vi "Example.vi"() -> ()   [LabVIEW 2023]
uses:
  BS6006PRPLUS.lvlib
panel:
  out "Serial Number":string
  in  "Pulse":u16(ring)=2 items=["-25 V  0.1 uJ DC-20 MHz", "-45 V  0.4 uJ  DC - 30 MHz", "-75 V  1.0 uJ  DC - 35 MHz", "-120 V  2.4 uJ  DC - 45 MHz", "-190 V  5.0 uJ  DC - 50 MHz", "-190 V  11 uJ  DC - 25 MHz", "-190 V  15 uJ  DC - 20 MHz", "-190 V  20 uJ  DC - 15 MHz", "-190 V  25 uJ  DC - 12 MHz", "-190 V  30 uJ  DC - 10 MHz", "-190 V  35 uJ  DC - 9 MHz", "-190 V  40 uJ  DC - 8 MHz", "-190 V  45 uJ  DC - 7 MHz", "-190 V  50 uJ  DC - 6 MHz"]
  in  "PRF (Hz)":u16(ring)=200 items=["100"=100, "200"=200, "500"=500, "1000"=1000, "2000"=2000, "5000"=5000, "10000"=10000]
  in  "End":bool
  out "Waveform Graph":dbl[][](graph)
  in  "Number of Signals to be Acquired":i32
  in  "Length of Signal":i32
  in  "Enable Waveform Acquisition":bool
  in  "Stop":bool
  in  "Run":bool
  in  "Trigger Source":u16(ring) items=["Internal", "External"]
  in  "Mode":u16(ring) items=["ECHO", "THRU"]
  in  "Gain":i32
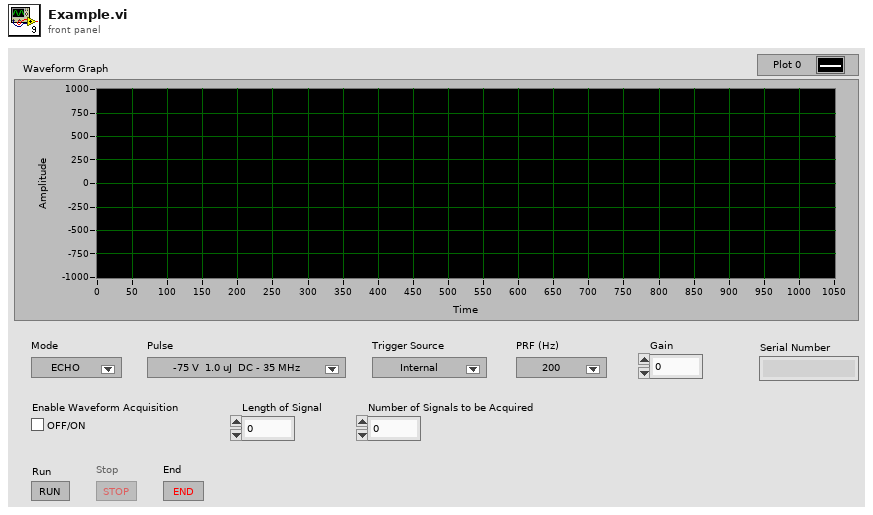
[diagram p1: front panel]
types:
  T1 = enum8{"Enabled", "Disabled", "Disabled and Grayed Out"}
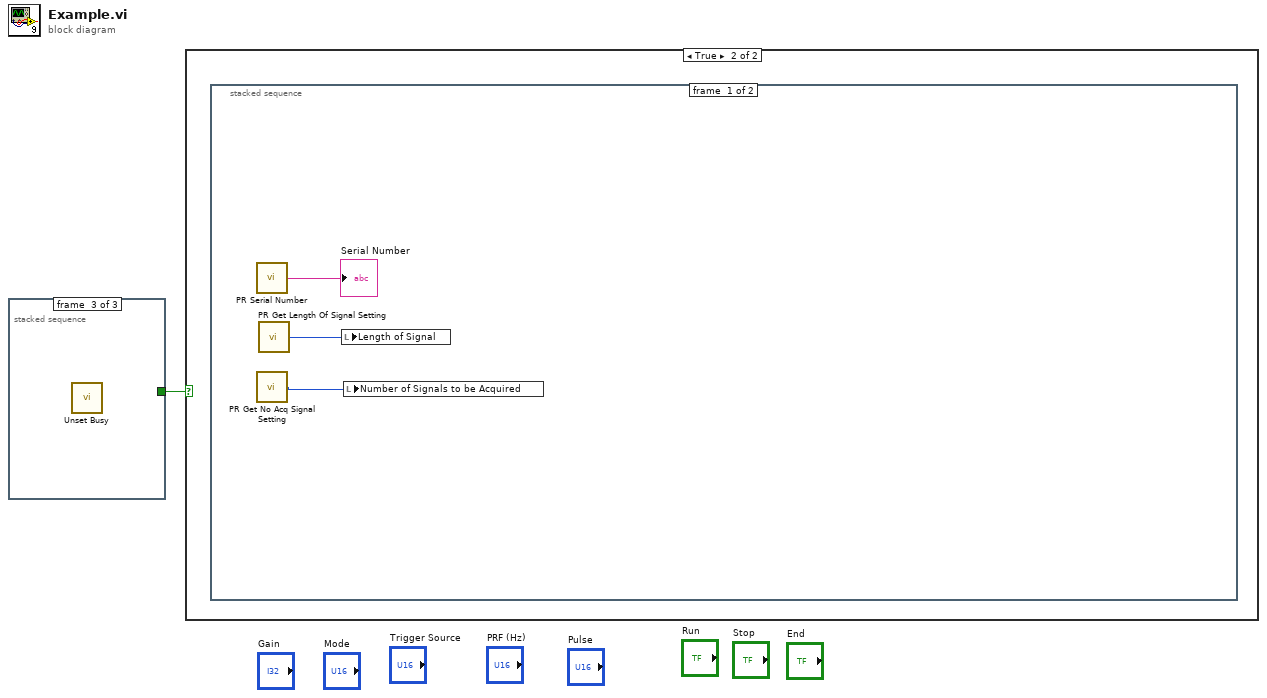
[diagram p0: block diagram]
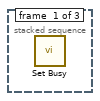
[diagram p2: hidden frame]
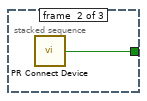
[diagram p3: hidden frame]
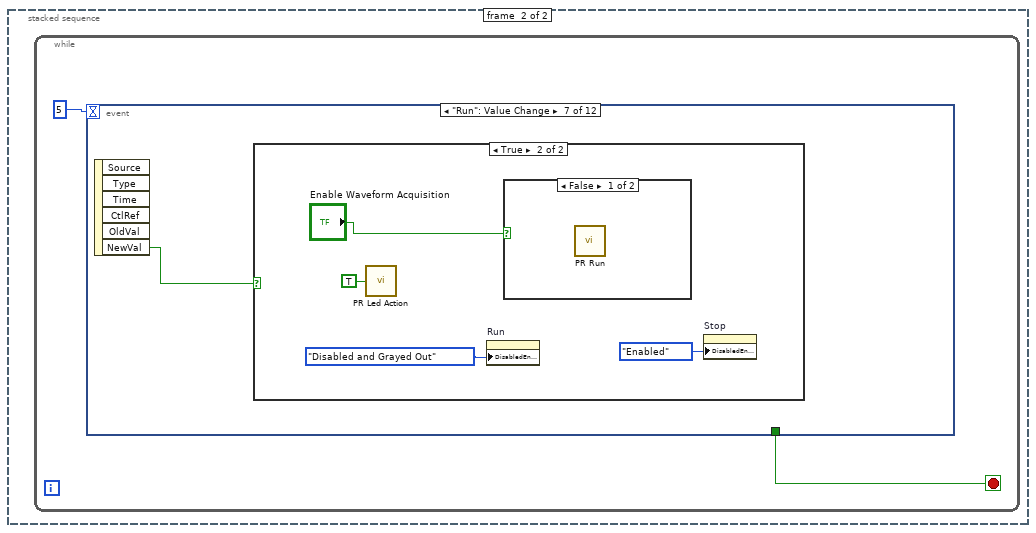
[diagram p5: hidden frame]
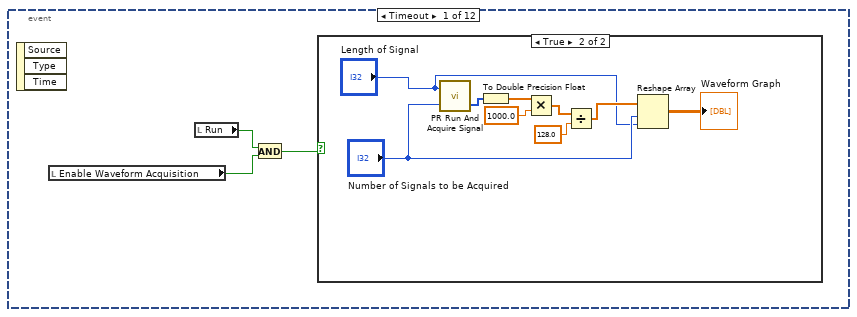
[diagram p6: hidden frame]
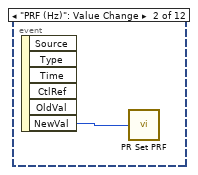
[diagram p8: hidden frame]
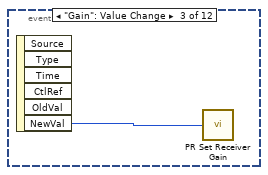
[diagram p9: hidden frame]
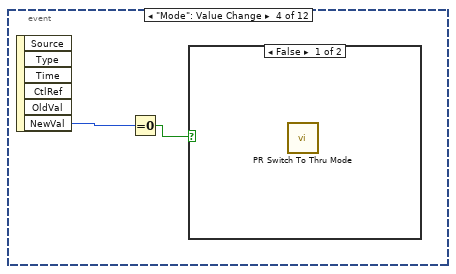
[diagram p10: hidden frame]
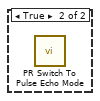
[diagram p11: hidden frame]
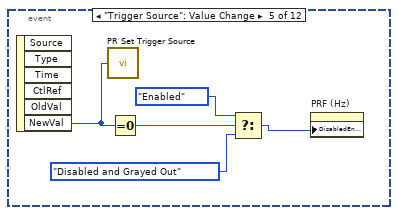
[diagram p12: hidden frame]
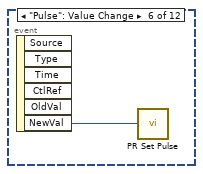
[diagram p13: hidden frame]
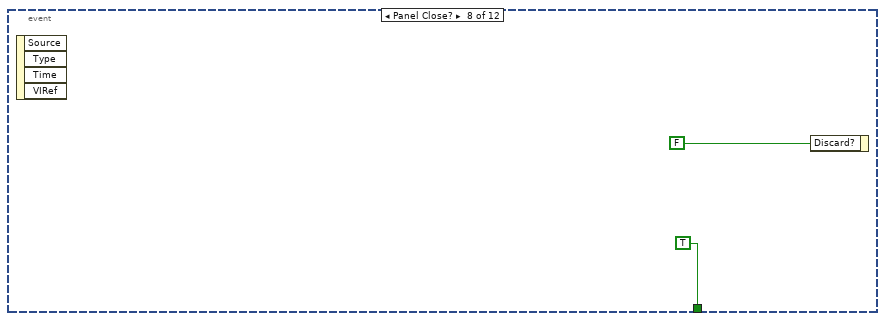
[diagram p16: hidden frame]
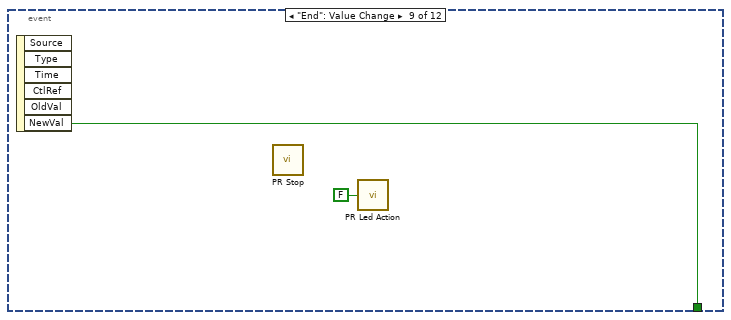
[diagram p17: hidden frame]
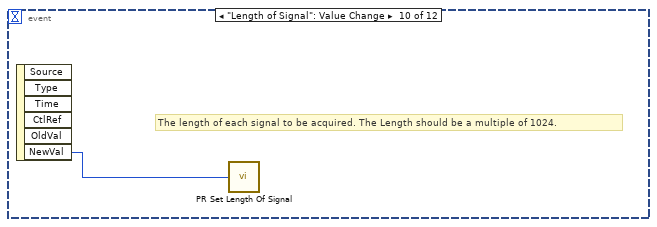
[diagram p18: hidden frame]
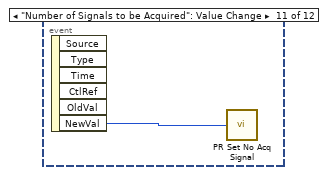
[diagram p19: hidden frame]
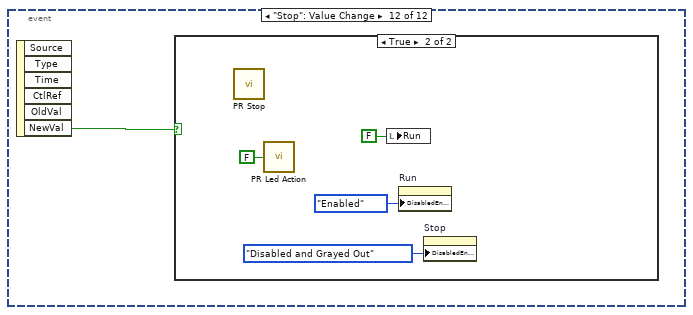
[diagram p20: hidden frame]
diagram:
  n1 = stacked-sequence {
    tunnel: [_ w2 _] -> w1
    frame #0 {
      n2 = call <vilib>:"Set Busy.vi"() -> ()  [unwired: 10 in, 2 out]
    }
    frame #1 {
      n3 = call "PR Connect Device.vi"() -> ("Connected"=w2:bool)
    }
    frame #2 {
      n4 = call <vilib>:"Unset Busy.vi"() -> ()  [unwired: 11 in, 1 out]
    }
  }
  n5 = case shown="True" w1 {
    frame False {
    }
    frame True {
      n6 = stacked-sequence {
        frame #0 {
          n7 = call "PR Serial Number.vi"() -> ("Serial Number"=→"Serial Number":string)
          n8 = call "PR Get No Acq Signal Setting.vi"() -> ("NoAcqSianglSetting"=w4:i32)
          n9 = call "PR Get Length Of Signal Setting.vi"() -> ("CurrentLength"=w5:i32)
          n10 = local write "Length of Signal"(w5) -> ()
          n11 = local write "Number of Signals to be Acquired"(w4) -> ()
        }
        frame #1 {
          n12 = while {
            stop <- w7 stop-if-true
            n13 = event shown="[6] \"Run\": Value Change" {
              selector: _ -> [_ _ _ _ _ _ _ _ _ _ _ _]
              dyn-events: _ -> [_ _ _ _ _ _ _ _ _ _ _ _]
              timeout: 5 -> [_ _ _ _ _ _ _ _ _ _ _ _]
              tunnel: [_ _ _ _ _ _ _ TRUE w38 _ _ _] -> w7
              event Timeout {
                n14 = event-data() -> ()  [unwired: 1 in, 3 out]
                n15 = local read "Enable Waveform Acquisition"() -> (w9:bool)
                n16 = local read "Run"() -> (w10:bool)
                n17 = And(x=w10, y=w9) -> (x .and. y?=w8:bool)
                n18 = case shown="True" w8 {
                  frame False {
                  }
                  frame True {
                    n19 = call "PR Run And Acquire Signal.vi"("Number of Signals to be Acquired"="Number of Signals to be Acquired", "Length of Signal"="Length of Signal") -> ("DataArray Out"=w19:i8[])  [unwired: 1 out]
                    n20 = To Double Precision Float(number=w19) -> (double precision float=w18:dbl[])
                    n21 = Multiply(x=w18, y=1000.0) -> (x*y=w16:dbl[])
                    n22 = Divide(x=w16, y=128.0) -> (x/y=w14:dbl[])
                    n23 = Reshape Array(w14, "Number of Signals to be Acquired", "Length of Signal") -> (→"Waveform Graph":dbl[][])
                  }
                }
              }
              event "PRF (Hz)": Value Change {
                n24 = event-data() -> ("NewVal"=w20:u16)  [unwired: 1 in, 5 out]
                n25 = call "PR Set PRF.vi"("PRF"=w20) -> ()  [unwired: 1 out]
              }
              event "Gain": Value Change {
                n26 = event-data() -> ("NewVal"=w21:i32)  [unwired: 1 in, 5 out]
                n27 = call "PR Set Receiver Gain.vi"("Gain"=w21) -> ()
              }
              event "Mode": Value Change {
                n28 = event-data() -> ("NewVal"=w23:u16)  [unwired: 1 in, 5 out]
                n29 = Equal To 0?(x=w23) -> (x = 0?=w22:bool)
                n30 = case shown="False" w22 {
                  frame False {
                    n31 = call "PR Switch To Thru Mode.vi"() -> ()  [unwired: 1 in]
                  }
                  frame True {
                    n32 = call "PR Switch To Pulse Echo Mode.vi"() -> ()  [unwired: 12 in]
                  }
                }
              }
              event "Trigger Source": Value Change {
                n33 = event-data() -> ("NewVal"=w28:u16)  [unwired: 1 in, 5 out]
                n34 = call "PR Set Trigger Source.vi"("TriggerSource"=w28) -> ()
                n35 = Equal To 0?(x=w28) -> (x = 0?=w27:bool)
                n36 = Select(t=T1."Enabled" ("Disabled"), s=w27, f=T1."Disabled and Grayed Out" ("Disabled")) -> (s? t:f=w24:T1)
                n37 = property on="PRF (Hz)" class="Ring (strict)"("DisabledEnum"=w24) -> ()  [unwired: 2 in, 2 out]
              }
              event "Pulse": Value Change {
                n38 = event-data() -> ("NewVal"=w29:u16)  [unwired: 1 in, 5 out]
                n39 = call "PR Set Pulse.vi"("PulseIndex"=w29) -> ()  [unwired: 1 out]
              }
              event "Run": Value Change {
                n40 = event-data() -> ("NewVal"=w30:bool)  [unwired: 1 in, 5 out]
                n41 = case shown="True" w30 {
                  frame False {
                  }
                  frame True {
                    n42 = call "PR Led Action.vi"("Enable"=TRUE) -> ()
                    n43 = property on="Run" class="Bool (strict)"("DisabledEnum"=T1."Disabled and Grayed Out" ("Disabled")) -> ()  [unwired: 2 in, 2 out]
                    n44 = case shown="False" "Enable Waveform Acquisition" {
                      frame False {
                        n45 = call "PR Run.vi"() -> ()  [unwired: 12 in]
                      }
                      frame True {
                      }
                    }
                    n46 = property on="Stop" class="Bool (strict)"("DisabledEnum"=T1."Enabled" ("Disabled")) -> ()  [unwired: 2 in, 2 out]
                  }
                }
              }
              event Panel Close? {
                n47 = event-data() -> ()  [unwired: 1 in, 4 out]
                n48 = event-data("Discard?"=FALSE) -> ()  [unwired: 1 in, 1 out]
              }
              event "End": Value Change {
                n49 = event-data() -> ("NewVal"=w38:bool)  [unwired: 1 in, 5 out]
                n50 = call "PR Stop.vi"() -> ()  [unwired: 12 in]
                n51 = call "PR Led Action.vi"("Enable"=FALSE) -> ()
              }
              event "Length of Signal": Value Change {
                # "The length of each signal to be acquired. The Length should be a multiple of 1024."
                n52 = event-data() -> ("NewVal"=w39:i32)  [unwired: 1 in, 5 out]
                n53 = call "PR Set Length Of Signal.vi"("Length"=w39) -> ()  [unwired: 1 out]
              }
              event "Number of Signals to be Acquired": Value Change {
                n54 = event-data() -> ("NewVal"=w40:i32)  [unwired: 1 in, 5 out]
                n55 = call "PR Set No Acq Signal.vi"("Number"=w40) -> ()  [unwired: 1 out]
              }
              event "Stop": Value Change {
                n56 = event-data() -> ("NewVal"=w41:bool)  [unwired: 1 in, 5 out]
                n57 = case shown="True" w41 {
                  frame False {
                  }
                  frame True {
                    n58 = call "PR Stop.vi"() -> ()  [unwired: 12 in]
                    n59 = call "PR Led Action.vi"("Enable"=FALSE) -> ()
                    n60 = local write "Run"(FALSE ("Run")) -> ()
                    n61 = property on="Run" class="Bool (strict)"("DisabledEnum"=T1."Enabled" ("Disabled")) -> ()  [unwired: 2 in, 2 out]
                    n62 = property on="Stop" class="Bool (strict)"("DisabledEnum"=T1."Disabled and Grayed Out" ("Disabled")) -> ()  [unwired: 2 in, 2 out]
                  }
                }
              }
            }
          }
        }
      }
    }
  }
